vi "MHM Get Config.vi"(8 "error in (no error)":errorcluster, 10 "ulConfig":u32, 11 "ulMHMHandle":u32) -> (0 "error out":errorcluster, 2 "pulValue":u32, 3 "function return":u32)   [LabVIEW 2019, in "MHM_1SL_interface.lvlib"]
uses:
  MHM_1SL_interface.lvlib
  lib/MHM_1SL_interface.dll
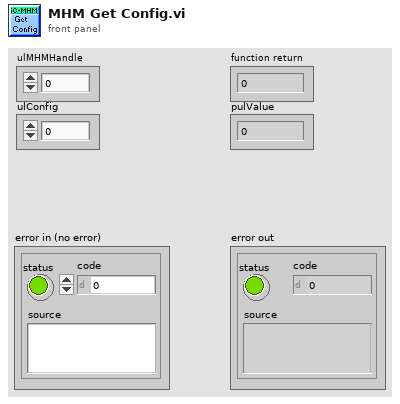
[diagram p1: front panel]
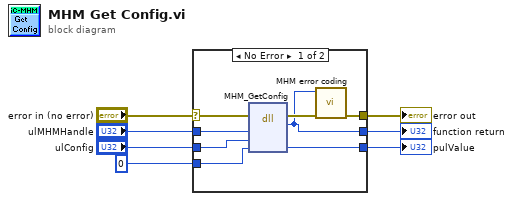
[diagram p0: block diagram]
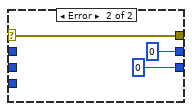
[diagram p2: hidden frame]
diagram:
  n1 = case shown="No Error" "error in (no error)" {
    selector: "error in (no error)" -> [w15 w18]
    tunnel: "ulMHMHandle" -> [w14 _]
    tunnel: "ulConfig" -> [w13 _]
    tunnel: u32 0 ("pulValue") -> [w12 _]
    tunnel: [w10 w18] -> w3
    tunnel: [w9 u32 0] -> w2
    tunnel: [w8 u32 0 ("pulValue")] -> w1
    frame No Error {
      n2 = dll-call lib="C:/workspace/project/scancon/MHM_1SL_interface_4.4.0/lv_interface/lib/MHM_1SL_interface.dll" fn="MHM_GetConfig"(error in=w15, "ulMHMHandle"=w14, "ulConfig"=w13, "pulValue"=w12) -> (error out=w11:errorcluster, "return type"=w9:u32, "pulValue"=w8:u32)  [unwired: 4 in, 1 out]
      n3 = call "MHM error coding.vi"("error in (no error)"=w11, "function return in"=w9) -> ("error out"=w10:errorcluster)  [unwired: 9 in]
    }
    frame Error {
    }
  }
  "function return" <- w2
  "pulValue" <- w1
  "error out" <- w3
